vi "SaveToFile.vi"(10 "FileNamePrefix":string="data", 11 "TextToWrite":string) -> ()   [LabVIEW 2018]
panel:
  out "error out":errorcluster
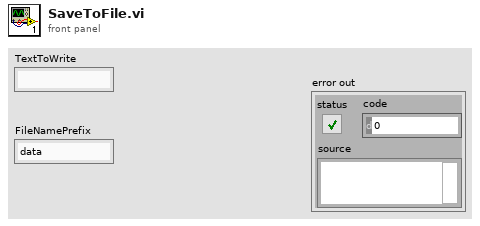
[diagram p1: front panel]
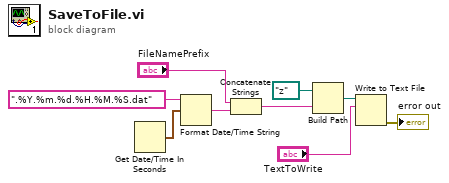
[diagram p0: block diagram]
diagram:
  n1 = Get Date/Time In Seconds() -> (seconds since 1Jan1904=w8:timestamp)
  n2 = Format Date/Time String(time format string (%c)=".%Y.%m.%d.%H.%M.%S.dat", seconds (now)=w8) -> (date/time string=w6:string)  [unwired: 1 in]
  n3 = Concatenate Strings("FileNamePrefix", w6) -> (w3:string)
  n4 = Build Path(base path=path "z:/", name or relative path=w3) -> (appended path=w1:path)
  n5 = Write to Text File(file (use dialog)=w1, text="TextToWrite") -> (error out=→"error out":errorcluster)  [unwired: 2 in, 2 out]
